vi "Flush.vi"(8 "error in (no error)":errorcluster, 11 "Queue in":refnum<queue>) -> (0 "error out":errorcluster, 1 "Data":string[](array[string]), 2 "Messages":string[](array[string]), 3 "Queue out":refnum<queue>, 4 "Elements":string[](array[string]))   [LabVIEW 2021, in "Queue.lvlib"]
doc: "Remove all elements in the queue. Returns the `<msg>,<data>` parts."
uses:
  Queue.lvlib
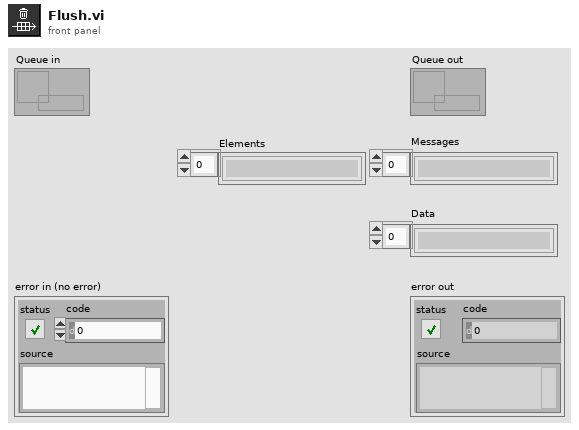
[diagram p1: front panel]
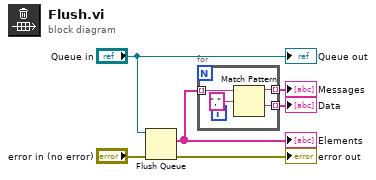
[diagram p0: block diagram]
diagram:
  n1 = Flush Queue(queue="Queue in", error in (no error)="error in (no error)") -> (remaining elements=w4:string[], error out=→"error out":errorcluster)  [unwired: 1 out]
  "Elements" <- w4
  n2 = for {
    tunnel: [w9] -> w6 mode=indexing
    tunnel: [w7] -> w5 mode=indexing
    tunnel: w4 -> [w8] mode=indexing
    n3 = Match Pattern(string=w8, regular expression=",") -> (before substring=w7:string, after substring=w9:string)  [unwired: 1 in, 2 out]
  }
  "Messages" <- w5
  "Data" <- w6
  "Queue out" <- "Queue in"
